vi "Send YIELD.vi"(8 "error in (no error)":errorcluster, 9 "Yield request":T1={"Invocation Request ID"=0, "Arguments"=[], "ArgumentsKw"="{}", "Options"="{}"}, 11 "WAMP Client in":refnum<class "WAMP Client.lvclass">) -> (0 "error out":errorcluster, 3 "WAMP Client out":refnum<class "WAMP Client.lvclass">)   [LabVIEW 2020, in "WAMP Client.lvclass"]
uses:
  <userlib>/wamplv/WAMP Client/WAMP Client.lvclass
  <userlib>/wamplv/WAMP Client/TypeDef/YIELD request data.ctl
  <userlib>/wamplv/WAMP Message Codes.ctl
  <userlib>/wamplv/WAMP Client/WAMP Client.lvclass/WAMP Client.ctl
  <vilib>/JDP Science/JSONtext/JSONtext.lvlib
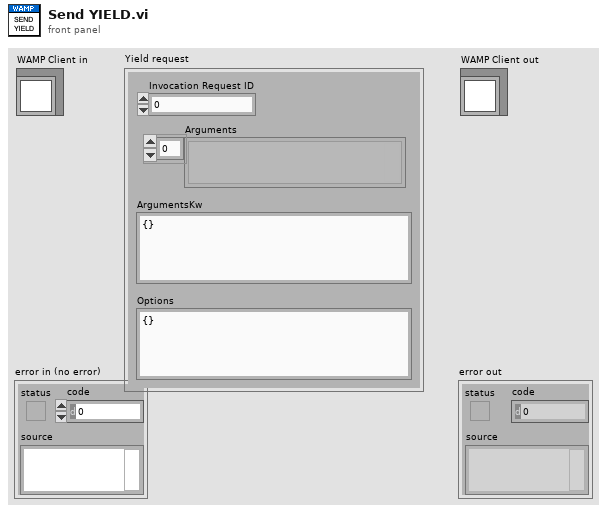
[diagram p1: front panel]
types:
  T1 = typedef "WAMP Client.lvclass/YIELD request data.ctl" = cluster{"Invocation Request ID":u32, "Arguments":variant[], "ArgumentsKw":string, "Options":string}
  T2 = typedef "WAMP Client.lvclass/WAMP Message Codes.ctl" = u16
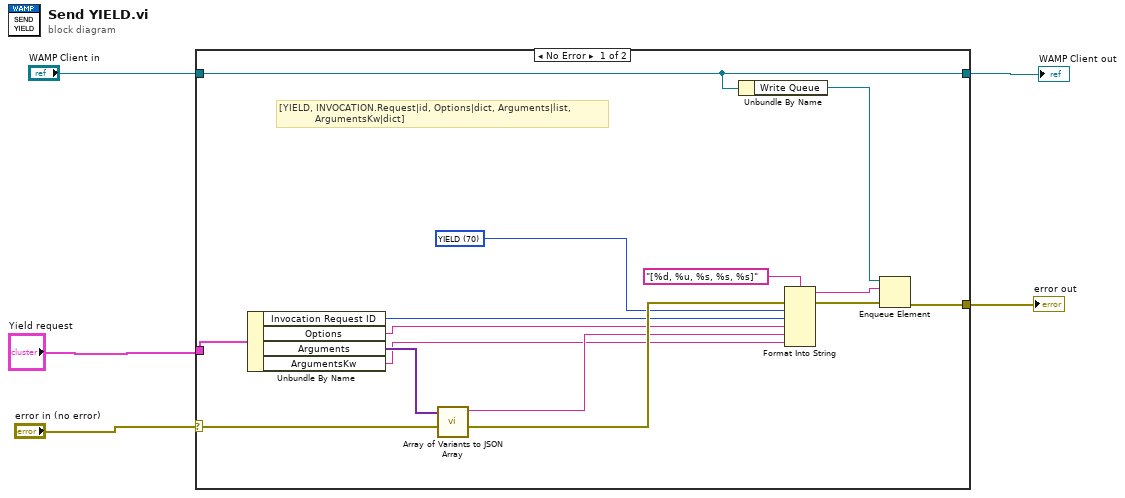
[diagram p0: block diagram]
diagram:
  n1 = case shown="No Error" "error in (no error)" {
    selector: "error in (no error)" -> [w15 w22]
    tunnel: [w20 w22] -> w4
    tunnel: [w13 w21] -> w2
    tunnel: "WAMP Client in" -> [w13 w21]
    tunnel: "Yield request" -> [w11 _]
    frame No Error {
      w12 = T2 70 items=["HELLO"=1, "WELCOME"=2, "ABORT"=3, "GOODBYE"=6, "ERROR"=8, "PUBLISH"=16, "PUBLISHED"=17, "SUBSCRIBE"=32, "SUBSCRIBED"=33, "UNSUBSCRIBE"=34, "UNSUBSCRIBED"=35, "EVENT"=36, "CALL"=48, "RESULT"=59, "REGISTER"=64, "REGISTERED"=65, "UNREGISTER"=66, "UNREGISTERED"=67, "INVOCATION"=68, "YIELD"=70] ("Message Codes")
      # "[YIELD, INVOCATION.Request|id, Options|dict, Arguments|list,\n            ArgumentsKw|dict]"
      n2 = Unbundle By Name(w11) -> ("Invocation Request ID"=w10:u32, "Options"=w9:string, "Arguments"=w8:variant[], "ArgumentsKw"=w6:string)
      n3 = call <vilib>:"Array of Variants to JSON Array.vi"("error in (no error)"=w15, "Array of Variants"=w8) -> ("error out"=w14:errorcluster, "<JSON>"=w7:string)  [unwired: 8 in]
      n4 = Unbundle By Name(w13) -> ("Write Queue"=w16:refnum<queue>)
      n5 = Format Into String(format string="[%d, %u, %s, %s, %s]" ("element"), error in=w14, w12, w10, w9, w7, w6) -> (resulting string=w18:string, error out=w17:errorcluster)  [unwired: 1 in]
      n6 = Enqueue Element(queue=w16, element=w18, error in (no error)=w17) -> (error out=w20:errorcluster)  [unwired: 1 in, 2 out]
    }
    frame Error {
    }
  }
  "error out" <- w4
  "WAMP Client out" <- w2
